vi "Add Modules from Configuration File.vi"(8 "error in (no error)":errorcluster, 10 "Configuration File Path":path, 11 "SLL Subpanel Manager in":refnum<class "SLL Subpanel Manager.lvclass">) -> (0 "error out":errorcluster, 3 "SLL Subpanel Manager out":refnum<class "SLL Subpanel Manager.lvclass">)   [LabVIEW 2014, in "SLL Subpanel Manager.lvclass"]
uses:
  SLL Subpanel Manager.lvclass
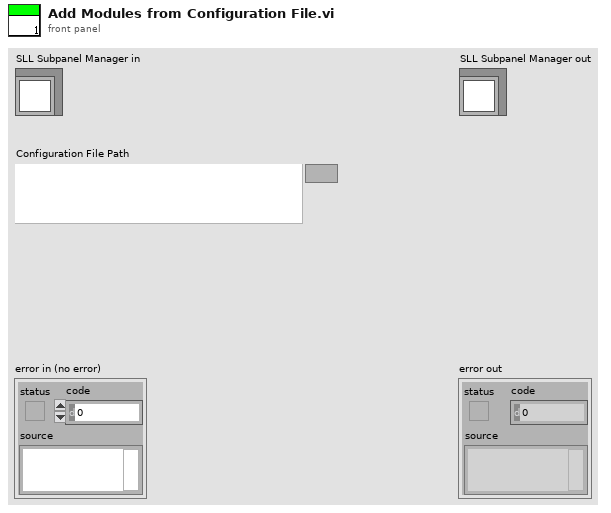
[diagram p1: front panel]
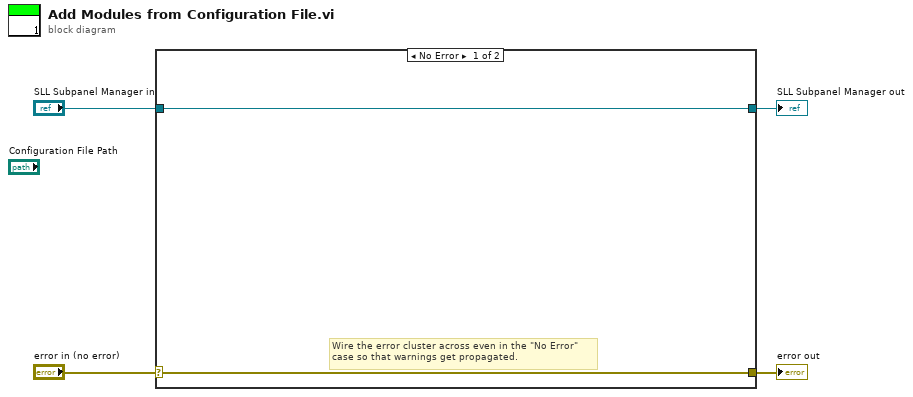
[diagram p0: block diagram]
diagram:
  n1 = case shown="No Error" "error in (no error)" {
    selector: "error in (no error)" -> [w6 w8]
    tunnel: [w6 w8] -> w3
    tunnel: [w5 w7] -> w1
    tunnel: "SLL Subpanel Manager in" -> [w5 w7]
    frame No Error {
      # "Wire the error cluster across even in the \"No Error\"\ncase so that warnings get propagated."
    }
    frame Error {
    }
  }
  "error out" <- w3
  "SLL Subpanel Manager out" <- w1
